vi "Read Return Address.vi"(11 "PreAddressedMsg in":refnum<class "PreAddressedMsg.lvclass">) -> (2 "Return Address":refnum<class "Message Enqueuer.lvclass">, 3 "PreAddressedMsg out":refnum<class "PreAddressedMsg.lvclass">)   [LabVIEW 2015, in "AbstractMessages.lvlib" / "PreAddressedMsg.lvclass"]
uses:
  PreAddressedMsg.lvclass
  <vilib>/ActorFramework/Message Enqueuer/Message Enqueuer.lvclass
  PreAddressedMsg.lvclass/PreAddressedMsg.ctl
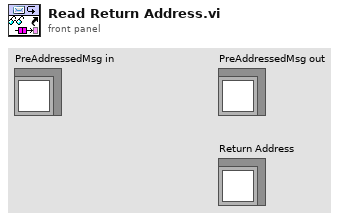
[diagram p1: front panel]
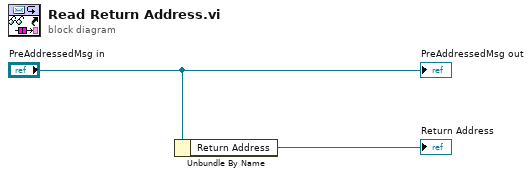
[diagram p0: block diagram]
diagram:
  n1 = Unbundle By Name("PreAddressedMsg in") -> ("Return Address"=→"Return Address":refnum<class "Message Enqueuer.lvclass">)
  "PreAddressedMsg out" <- "PreAddressedMsg in"
